vi "Create.vi"() -> (8 "Pulse Train":refnum<class "Pulse Train.lvclass">)   [LabVIEW 2020, in "Pulse Train.lvclass"]
uses:
  Pulse Train.lvclass
  Pulse Train.lvclass/Pulse Train.ctl
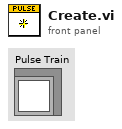
[diagram p1: front panel]
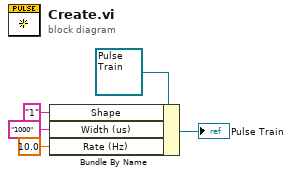
[diagram p0: block diagram]
diagram:
  n1 = Bundle By Name(cluster=refnum<class "Pulse Train.lvclass"> refnum ("Pulse Train"), "Shape"="1" ("Serialized.Shape"), "Width (us)"="1000" ("Serialized.Width (us)"), "Rate (Hz)"=10.0 ("Serialized.Rate (Hz)")) -> (→"Pulse Train":refnum<class "Pulse Train.lvclass">)
